vi "Build Love.vi"(11 "N":i32) -> (3 "Graph":cluster{dbl[], dbl[]})   [LabVIEW 2015]
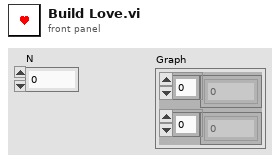
[diagram p1: front panel]
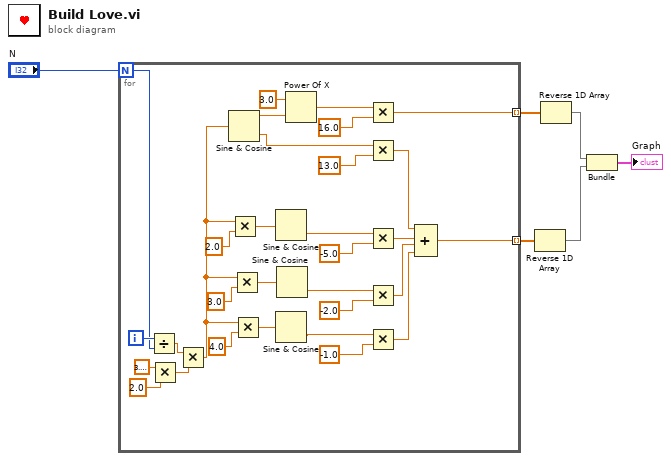
[diagram p0: block diagram]
diagram:
  n1 = for {
    N: "N" -> [w9]
    tunnel: [w8] -> w4 mode=indexing
    tunnel: [w7] -> w5 mode=indexing
    i -> [w37]
    n2 = Divide(x=w37, y=w9) -> (x/y=w11:dbl)
    n3 = Multiply(x=3.141592653589793, y=2.0) -> (x*y=w12:dbl)
    n4 = Multiply(x=w11, y=w12) -> (x*y=w10:dbl)
    n5 = Sine & Cosine(0:w10) -> (1:w36:dbl, 2:w31:dbl)
    n6 = Multiply(x=w10, y=2.0) -> (x*y=w27:dbl)
    n7 = Multiply(x=w10, y=3.0) -> (x*y=w26:dbl)
    n8 = Multiply(x=w10, y=4.0) -> (x*y=w25:dbl)
    n9 = Sine & Cosine(0:w27) -> (2:w23:dbl)  [unwired: 1 out]
    n10 = Sine & Cosine(0:w25) -> (2:w19:dbl)  [unwired: 1 out]
    n11 = Sine & Cosine(0:w26) -> (2:w21:dbl)  [unwired: 1 out]
    n12 = Power Of X(1:w36, 2:3.0 ("y")) -> (0:w34:dbl)
    n13 = Multiply(x=w34, y=16.0) -> (x*y=w8:dbl)
    n14 = Multiply(x=w31, y=13.0) -> (x*y=w16:dbl)
    n15 = Multiply(x=w23, y=-5.0) -> (x*y=w18:dbl)
    n16 = Multiply(x=w21, y=-2.0) -> (x*y=w17:dbl)
    n17 = Multiply(x=w19, y=-1.0) -> (x*y=w15:dbl)
    n18 = Compound Arithmetic op=ADD(w16, w18, w17, w15) -> (w7:dbl)
  }
  n19 = Reverse 1D Array(array=w5) -> (reversed array=w1:dbl[])
  n20 = Reverse 1D Array(array=w4) -> (reversed array=w2:dbl[])
  n21 = Bundle(w2, w1) -> (→"Graph":cluster{dbl[], dbl[]})  [unwired: 1 in]
